vi "PrintHello.vi"(8 "error in (no error)":errorcluster, 11 "ProductA in":refnum<class "ProductA.lvclass">) -> (0 "error out":errorcluster, 3 "ProductA out":refnum<class "ProductA.lvclass">)   [LabVIEW 2017, in "ProductA.lvclass"]
uses:
  ProductA.lvclass
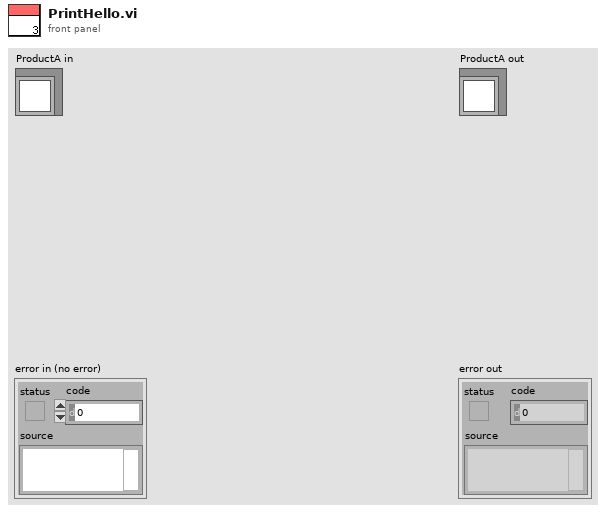
[diagram p1: front panel]
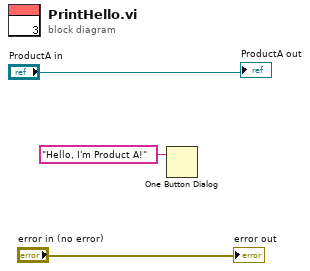
[diagram p0: block diagram]
diagram:
  n1 = One Button Dialog(message="Hello, I'm Product A!") -> ()  [unwired: 1 in, 1 out]
  "error out" <- "error in (no error)"
  "ProductA out" <- "ProductA in"
